vi "ep_Get Gain Calibrations Points.vi"(0 "Calibration":T1={"voltage"={"full-range RMS values"=[5.0, 5.0, 5.0], "time domain"={"ranges to calibrate [%]"=[100.0], "offsets"=[0.0, 0.0, 0.0], "gains"=[[1.0], [1.0], [1.0]]}, "frequency domain"={"ranges to calibrate [%]"=[100.0], "frequencies to calibrate [Hz]"=[50.0], "phase delays [deg]"=[[[0.0]], [[0.0]], [[0.0]]], "gains"=[[[1.0]], [[1.0]], [[1.0]]]}}, "current"={"full-range RMS values"=[300.0, 300.0, 300.0, 300.0], "time domain"={"ranges to calibrate [%]"=[100.0], "offsets"=[0.0, 0.0, 0.0, 0.0], "gains"=[[1.0], [1.0], [1.0], [1.0]]}, "frequency domain"={"ranges to calibrate [%]"=[100.0], "frequencies to calibrate [Hz]"=[50.0], "phase delays [deg]"=[[[0.0]], [[0.0]], [[0.0]], [[0.0]]], "gains"=[[[1.0]], [[1.0]], [[1.0]], [[1.0]]]}}}) -> (4 "voltages#":i32, 6 "voltages RMS":dbl[](array[numeric]), 8 "currents RMS":dbl[](array[numeric]))   [LabVIEW 2012]
uses:
  <vilib>/addons/Electrical Power/Example Support/PQ/Calibration/ep_Calibration.ctl
panel:
  out "RMS":dbl[](array[numeric])
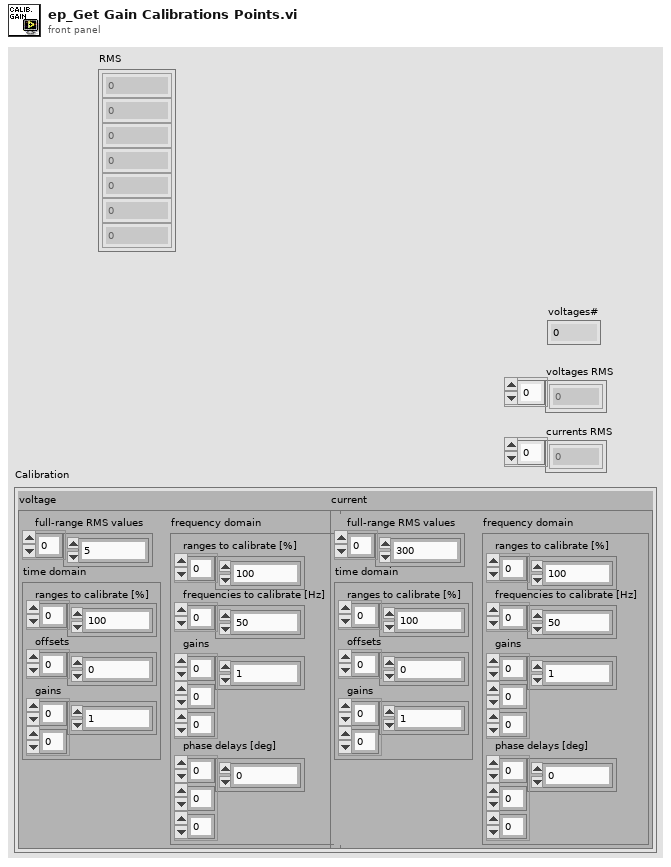
[diagram p1: front panel]
types:
  T1 = typedef "ep_Calibration.ctl" = cluster{"voltage":cluster{"full-range RMS values":dbl[], "time domain":cluster{"ranges to calibrate [%]":dbl[], "offsets":dbl[], "gains":dbl[][]}, "frequency domain":cluster{"ranges to calibrate [%]":dbl[], "frequencies to calibrate [Hz]":dbl[], "phase delays [deg]":dbl[][][], "gains":dbl[][][]}}, "current":cluster{"full-range RMS values":dbl[], "time domain":cluster{"ranges to calibrate [%]":dbl[], "offsets":dbl[], "gains":dbl[][]}, "frequency domain":cluster{"ranges to calibrate [%]":dbl[], "frequencies to calibrate [Hz]":dbl[], "phase delays [deg]":dbl[][][], "gains":dbl[][][]}}}
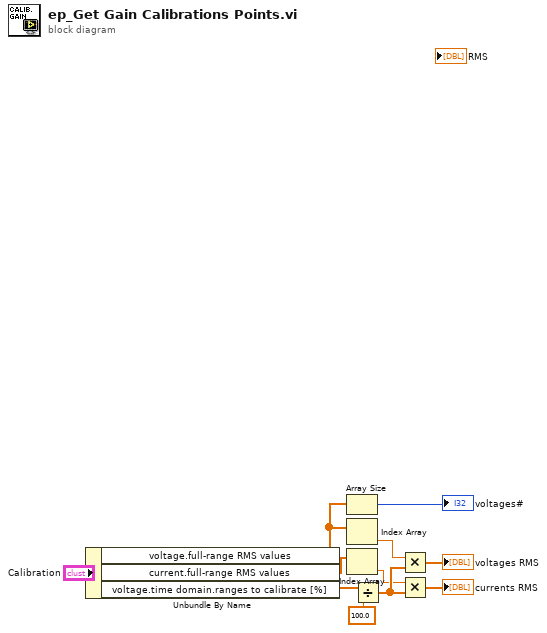
[diagram p0: block diagram]
diagram:
  n1 = Unbundle By Name("Calibration") -> ("voltage.full-range RMS values"=w4:dbl[], "current.full-range RMS values"=w2:dbl[], "voltage.time domain.ranges to calibrate [%]"=w8:dbl[])
  n2 = Array Size(array=w4) -> (size(s)=→"voltages#":i32)
  n3 = Index Array(array=w4) -> (element=w3:dbl)  [unwired: 1 in]
  n4 = Index Array(array=w2) -> (element=w1:dbl)  [unwired: 1 in]
  n5 = Divide(x=w8, y=100.0 ("element")) -> (x/y=w10:dbl[])
  n6 = Multiply(x=w3, y=w10) -> (x*y=→"voltages RMS":dbl[])
  n7 = Multiply(x=w1, y=w10) -> (x*y=→"currents RMS":dbl[])
